vi "Initial MovCor-format and values.vi"() -> (14 "Ini file interface (DBL)":T3, 15 "DBL values":dbl[](array[numeric]), 16 "String":T1, 17 "String values":string[](array[string]), 18 "Boolean":T2, 19 "Boolean values":bool[](array[boolean]))   [LabVIEW 2020]
uses:
  Typedefs/Ini file interface (DBL).ctl
  Typedefs/Ini file interface (Boolean).ctl
  Typedefs/Ini file interface (String).ctl
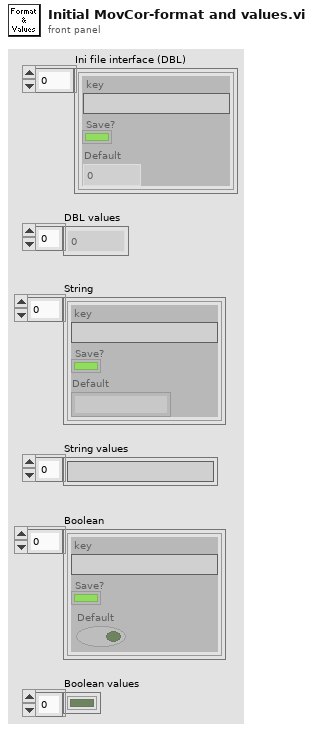
[diagram p1: front panel]
types:
  T1 = typedef "Ini file interface (String).ctl" = cluster{"key":string, "Save?":bool, "Default":string}[]
  T2 = typedef "Ini file interface (Boolean).ctl" = cluster{"key":string, "Save?":bool, "Default":bool}[]
  T3 = typedef "Ini file interface (DBL).ctl" = cluster{"key":string, "Save?":bool, "Default":dbl}[]
  T4 = typedef "Ref DAQ Param.ctl" = cluster{"Full Frame Size":u16, "Ref Field of View":sgl, "Ref Zoom":i8, "Ref_dwellTime":sgl, "Ref X-pixels-per-line(Npxr)":i16, "Ref Y-lines-per-image(Npyr)":i16, "Ref Z-lines-per-image":i16, "Ignore Z lines":i16, "Ref Scan Cycles":i32, "Ref threshold XY":u16, "Ref threshold Z":u16, "Ref average XY":u16, "Ref Average  Z":u16, "Proportional_scale":fxp<+,16,2>, "Integral_scale":fxp<+/-,16,12>, "Proportional_scale Z":fxp<+,16,2>, "Integral_scale Z":fxp<+/-,16,12>, "Diff_threshold":fxp<+,16,2>, "Diff_threshold _z":fxp<+,16,2>, "Sliding Average":bool, "Ref count reset enabled":bool}
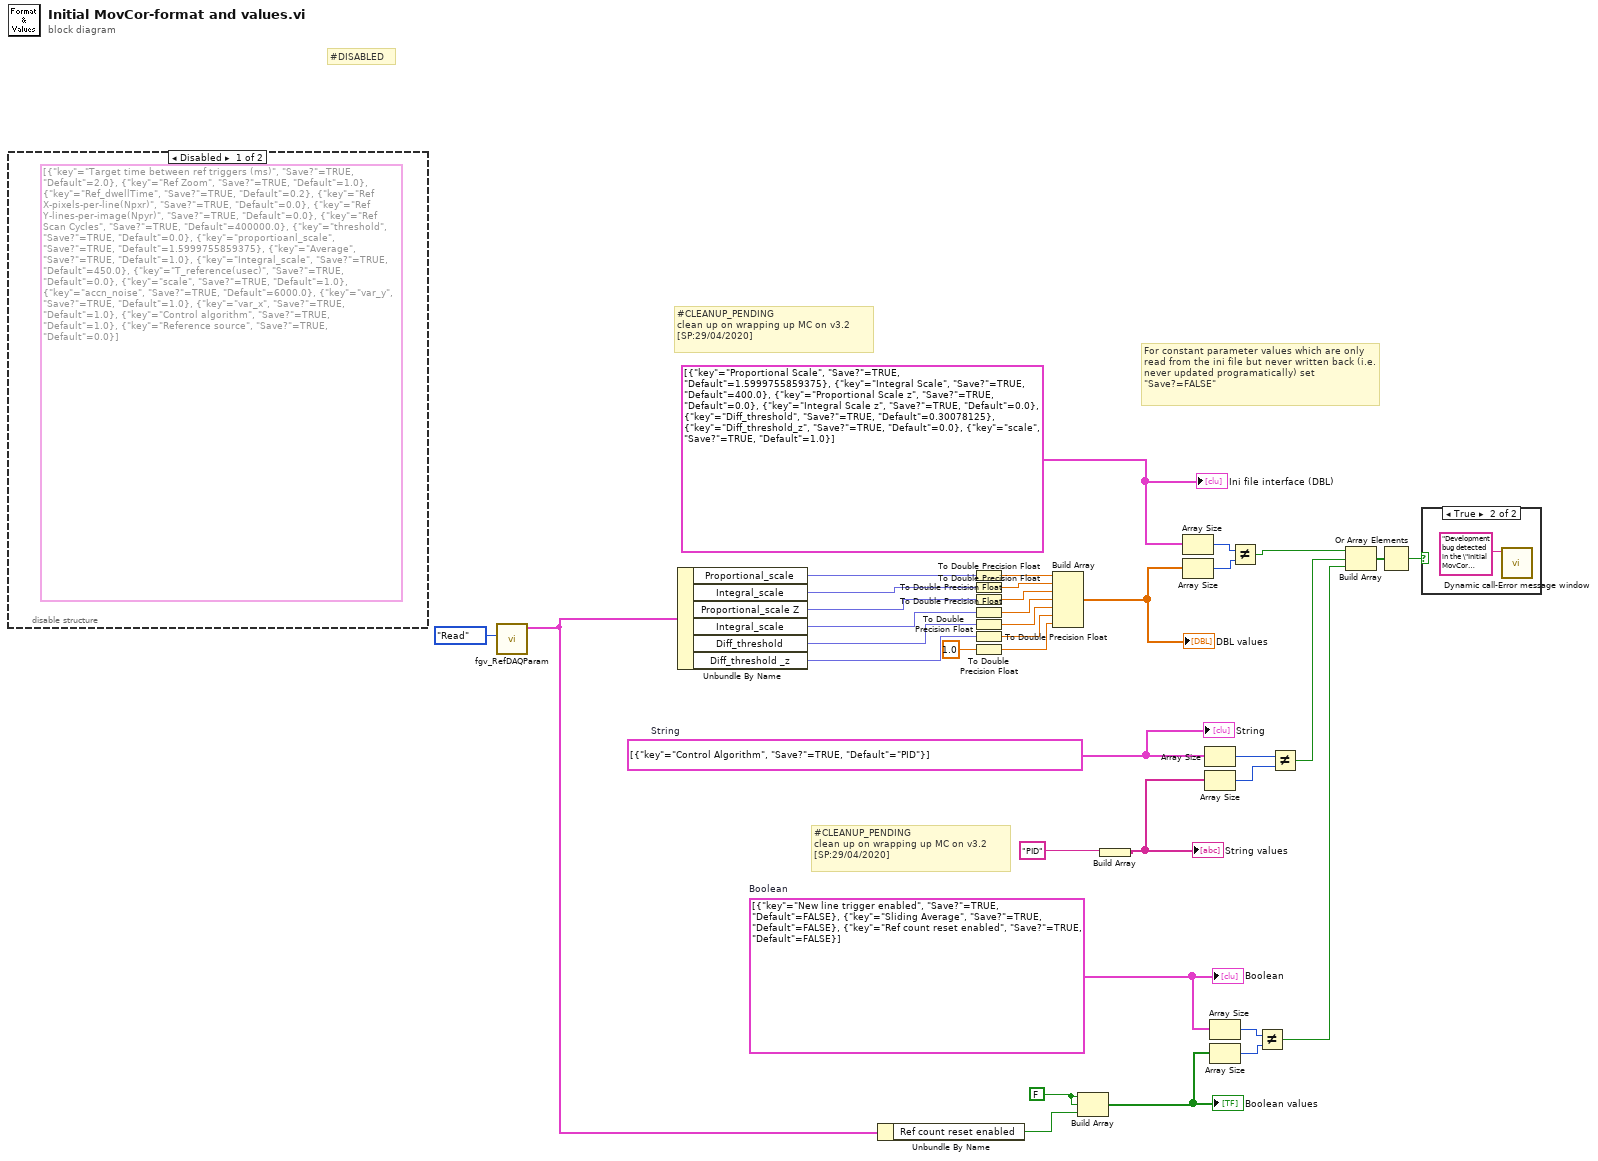
[diagram p0: block diagram]
diagram:
  w2 = FALSE ("element")
  w31 = T3 [{"key"="Proportional Scale", "Save?"=TRUE, "Default"=1.5999755859375}, {"key"="Integral Scale", "Save?"=TRUE, "Default"=400.0}, {"key"="Proportional Scale z", "Save?"=TRUE, "Default"=0.0}, {"key"="Integral Scale z", "Save?"=TRUE, "Default"=0.0}, {"key"="Diff_threshold", "Save?"=TRUE, "Default"=0.30078125}, {"key"="Diff_threshold_z", "Save?"=TRUE, "Default"=0.0}, {"key"="scale", "Save?"=TRUE, "Default"=1.0}] ("Ini file interface (DBL)")
  w23 = T2 [{"key"="New line trigger enabled", "Save?"=TRUE, "Default"=FALSE}, {"key"="Sliding Average", "Save?"=TRUE, "Default"=FALSE}, {"key"="Ref count reset enabled", "Save?"=TRUE, "Default"=FALSE}]  # Boolean
  w27 = T1 [{"key"="Control Algorithm", "Save?"=TRUE, "Default"="PID"}]  # String
  # "#CLEANUP_PENDING\nclean up on wrapping up MC on v3.2\n[SP:29/04/2020]"
  # "#CLEANUP_PENDING\nclean up on wrapping up MC on v3.2\n[SP:29/04/2020]"
  # "#DISABLED"
  # "For constant parameter values which are only read from the ini file but never written back (i.e. never updated programatically) set \"Save?=FALSE\""
  n1 = disable-structure shown="Disabled" {
    frame Disabled {
      (unwired) T3 [{"key"="Target time between ref triggers (ms)", "Save?"=TRUE, "Default"=2.0}, {"key"="Ref Zoom", "Save?"=TRUE, "Default"=1.0}, {"key"="Ref_dwellTime", "Save?"=TRUE, "Default"=0.2}, {"key"="Ref X-pixels-per-line(Npxr)", "Save?"=TRUE, "Default"=0.0}, {"key"="Ref Y-lines-per-image(Npyr)", "Save?"=TRUE, "Default"=0.0}, {"key"="Ref Scan Cycles", "Save?"=TRUE, "Default"=400000.0}, {"key"="threshold", "Save?"=TRUE, "Default"=0.0}, {"key"="proportioanl_scale", "Save?"=TRUE, "Default"=1.5999755859375}, {"key"="Average", "Save?"=TRUE, "Default"=1.0}, {"key"="Integral_scale", "Save?"=TRUE, "Default"=450.0}, {"key"="T_reference(usec)", "Save?"=TRUE, "Default"=0.0}, {"key"="scale", "Save?"=TRUE, "Default"=1.0}, {"key"="accn_noise", "Save?"=TRUE, "Default"=6000.0}, {"key"="var_y", "Save?"=TRUE, "Default"=1.0}, {"key"="var_x", "Save?"=TRUE, "Default"=1.0}, {"key"="Control algorithm", "Save?"=TRUE, "Default"=1.0}, {"key"="Reference source", "Save?"=TRUE, "Default"=0.0}] ("Ini file interface (DBL)")
    }
    frame Enabled {
    }
  }
  n2 = call "fgv_RefDAQParam.vi"("Function"=enum16{"Initialize", "Write", "Read"}."Read") -> ("RefDAQParam"=w20:T4)  [unwired: 9 in, 1 out]
  n3 = Unbundle By Name(w20) -> ("Proportional_scale"=w17:fxp<+,16,2>, "Integral_scale"=w16:fxp<+/-,16,12>, "Proportional_scale Z"=w15:fxp<+,16,2>, "Integral_scale"=w14:fxp<+/-,16,12>, "Diff_threshold"=w13:fxp<+,16,2>, "Diff_threshold _z"=w12:fxp<+,16,2>)
  n4 = Unbundle By Name(w20) -> ("Ref count reset enabled"=w3:bool)
  n5 = To Double Precision Float(number=w17) -> (double precision float=w11:dbl)
  n6 = To Double Precision Float(number=w16) -> (double precision float=w10:dbl)
  n7 = To Double Precision Float(number=w15) -> (double precision float=w9:dbl)
  n8 = To Double Precision Float(number=w14) -> (double precision float=w8:dbl)
  n9 = To Double Precision Float(number=w13) -> (double precision float=w7:dbl)
  n10 = To Double Precision Float(number=w12) -> (double precision float=w6:dbl)
  n11 = To Double Precision Float(number=1.0) -> (double precision float=w5:dbl)
  n12 = Build Array(w11, w10, w9, w8, w7, w6, w5) -> (w4:dbl[])
  "DBL values" <- w4
  n13 = Build Array(w2, w2, w3) -> (w22:bool[])
  "Boolean values" <- w22
  n14 = Build Array("PID") -> (w18:string[])
  "String values" <- w18
  n15 = Array Size(array=w31) -> (size(s)=w35:i32)
  n16 = Array Size(array=w4) -> (size(s)=w34:i32)
  n17 = Array Size(array=w27) -> (size(s)=w28:i32)
  n18 = Array Size(array=w18) -> (size(s)=w29:i32)
  n19 = Array Size(array=w23) -> (size(s)=w25:i32)
  n20 = Array Size(array=w22) -> (size(s)=w24:i32)
  n21 = Not Equal?(x=w35, y=w34) -> (x != y?=w30:bool)
  n22 = Not Equal?(x=w25, y=w24) -> (x != y?=w21:bool)
  n23 = Not Equal?(x=w28, y=w29) -> (x != y?=w26:bool)
  n24 = Build Array(w30, w26, w21) -> (w33:bool[])
  n25 = Or Array Elements(Boolean array=w33) -> (logical OR=w32:bool)
  n26 = case shown="True" w32 {
    frame False {
    }
    frame True {
      n27 = call "Dynamic call-Error message window.vi"("Error Message"="Development bug detected in the \"Initial MovCor parser.vi\"\nPlease correct the set up in this VI.") -> ()  [unwired: 10 in, 1 out]
    }
  }
  "Ini file interface (DBL)" <- w31
  "Boolean" <- w23
  "String" <- w27
